vi "DblToStrForAcquire.vi"(11 "DataDbl":dbl[](array[numeric])=[0.00234, 2.0, 3.0, 4.0]) -> (3 "Out":string[](array[string])=["2.340E-3", "2.000E+0", "3.000E+0", "4.000E+0"])   [LabVIEW 2017]
panel:
  in  "Out 2":string[](array[string])=["%^.0f", "%^.5f", "%^.5f", "%^.5f"]
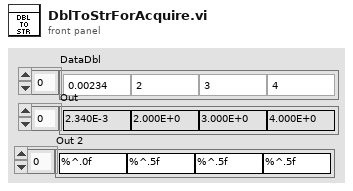
[diagram p1: front panel]
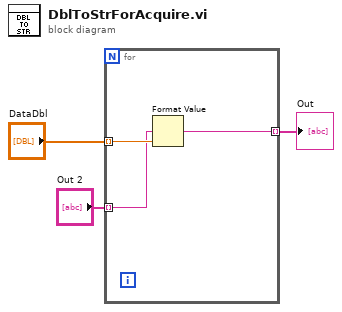
[diagram p0: block diagram]
diagram:
  n1 = for {
    tunnel: "DataDbl" -> [w6] mode=indexing
    tunnel: [w5] -> w2 mode=indexing
    tunnel: "Out 2" -> [w4] mode=indexing
    n2 = Format Value(format string=w4, value (0)=w6) -> (output string=w5:string)  [unwired: 1 in]
  }
  "Out" <- w2
